vi "InitializeKeithley6485.vi"(8 "Error In":errorcluster, 10 "Keithley 6485":T1, 11 "VISA Resources":string[](array[string])) -> (0 "Error Out":errorcluster, 3 "Keithley 6485 Out":refnum<visa-resource-name>[](array[refnum]))   [LabVIEW 2012]
uses:
  Keithley6485Configuration.ctl
  libs/Keithley-6485/Public/Controls/FormatElement.ctl
  libs/Keithley-6485/Public/Controls/DataFormat.ctl
  libs/Keithley-6485/Keithley-6485.lvlib
  libs/LV-Utilities/LV-Utilities.lvlib
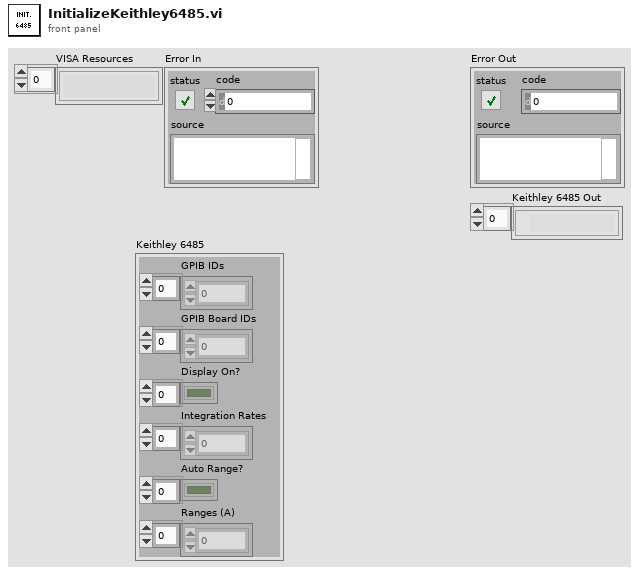
[diagram p1: front panel]
types:
  T1 = typedef "Keithley6485Configuration.ctl" = cluster{"GPIB IDs":u8[], "GPIB Board IDs":u8[], "Display On?":bool[], "Integration Rates":dbl[], "Auto Range?":bool[], "Ranges (A)":dbl[]}
  T2 = typedef "Keithley-6485.lvlib/DataFormat.ctl" = enum16{"ASCII", "Real", "32", "Sreal"}
  T3 = typedef "Keithley-6485.lvlib/FormatElement.ctl" = enum16{"Read", "Unit", "Time", "Status"}
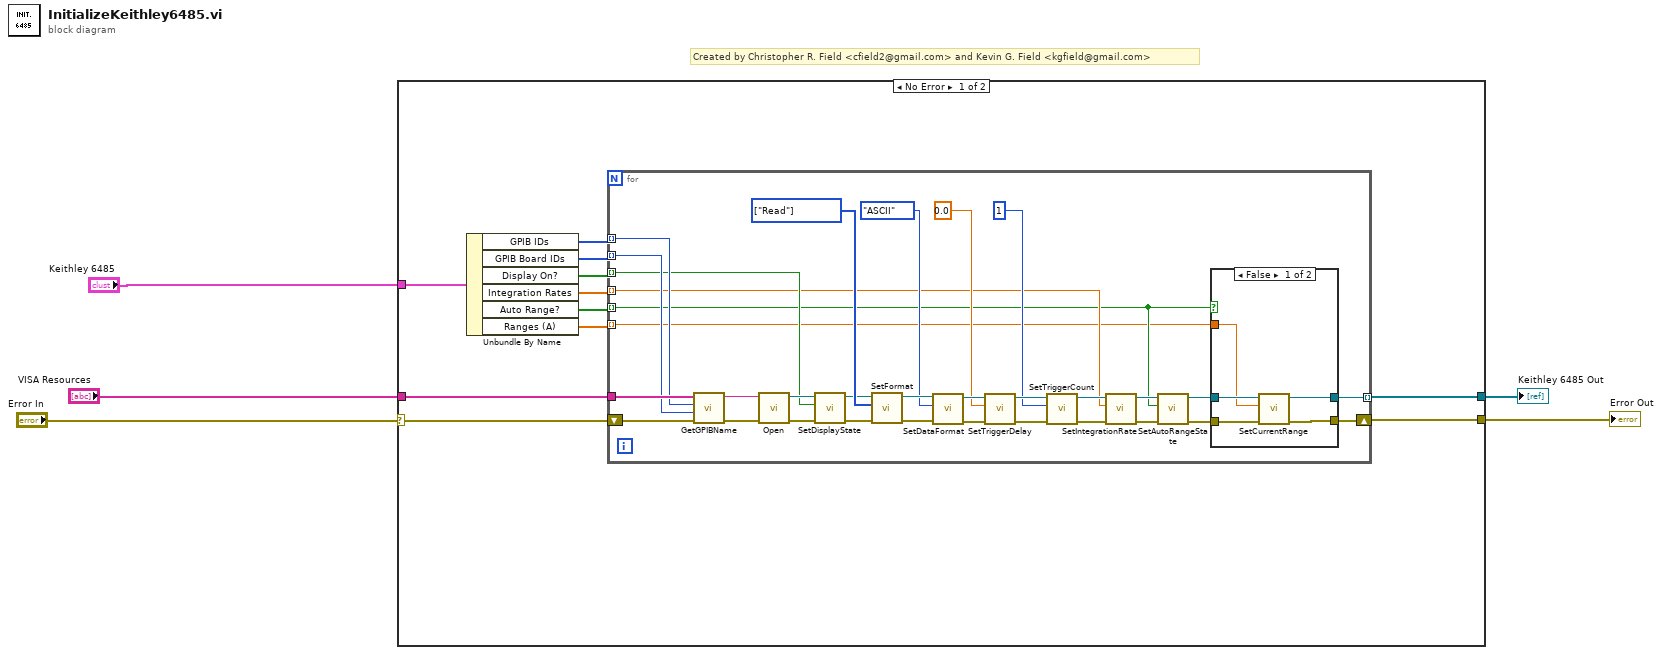
[diagram p0: block diagram]
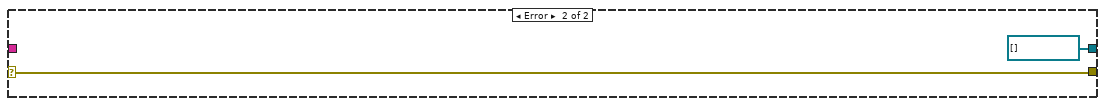
[diagram p3: hidden frame]
diagram:
  # "Created by Christopher R. Field <cfield2@gmail.com> and Kevin G. Field <kgfield@gmail.com>"
  n1 = case shown="No Error" "Error In" {
    selector: "Error In" -> [w6 w57]
    tunnel: "Keithley 6485" -> [w16 _]
    tunnel: "VISA Resources" -> [w9 _]
    tunnel: [w8 w57] -> w3
    tunnel: [w7 refnum<visa-resource-name>[] []] -> w2
    frame No Error {
      n2 = Unbundle By Name(w16) -> ("GPIB IDs"=w15:u8[], "GPIB Board IDs"=w14:u8[], "Display On?"=w13:bool[], "Integration Rates"=w12:dbl[], "Auto Range?"=w11:bool[], "Ranges (A)"=w10:dbl[])
      n3 = for {
        tunnel: w9 -> [w48]
        tunnel: w15 -> [w47] mode=indexing
        tunnel: w14 -> [w46] mode=indexing
        tunnel: w13 -> [w41] mode=indexing
        tunnel: [w19] -> w7 mode=indexing
        shift-right: [w18] -> w8
        shift-left: w6 -> [w24]
        tunnel: w12 -> [w23] mode=indexing
        tunnel: w11 -> [w22] mode=indexing
        tunnel: w10 -> [w17] mode=indexing
        w40 = T3[] [enum."Read"] items=["Read", "Unit", "Time", "Status"] ("Format Elements")
        n4 = call "GetGPIBName.vi"("Error In"=w24, "GPIB ID"=w46, "GPIB Board"=w47, "VISA Resource List"=w48) -> ("Error Out"=w45:errorcluster, "VISA GPIB Resource Name"=w44:string)  [unwired: 5 in, 1 out]
        n5 = call "Open.vi"("Error In"=w45, "Keithley 6485 In"=w44) -> ("Error Out"=w42:errorcluster, "Keithley 6485 Out"=w43:refnum<visa-resource-name>)  [unwired: 8 in]
        n6 = call "SetDisplayState.vi"("Error In"=w42, "Enabled?"=w41, "Keithley 6485 In"=w43) -> ("Error Out"=w38:errorcluster, "Keithley 6485 Out"=w39:refnum<visa-resource-name>)  [unwired: 7 in]
        n7 = call "SetFormat.vi"("Error In"=w38, "Format Elements"=w40, "Keithley 6485 In"=w39) -> ("Error Out"=w36:errorcluster, "Keithley 6485 Out"=w37:refnum<visa-resource-name>)  [unwired: 7 in]
        n8 = call "SetDataFormat.vi"("Error In"=w36, "Data Format"=DataFormat."ASCII", "Keithley 6485 In"=w37) -> ("Error Out"=w33:errorcluster, "Keithley 6485 Out"=w34:refnum<visa-resource-name>)  [unwired: 7 in]
        n9 = call "SetTriggerDelay.vi"("Error In"=w33, "Delay (sec)"=0.0, "Keithley 6485 In"=w34) -> ("Error Out"=w30:errorcluster, "Keithley 6485 Out"=w31:refnum<visa-resource-name>)  [unwired: 7 in]
        n10 = call "SetTriggerCount.vi"("Error In"=w30, "Count (1-3000)"=u16 1, "Keithley 6485 In"=w31) -> ("Error Out"=w27:errorcluster, "Keithley 6485 Out"=w28:refnum<visa-resource-name>)  [unwired: 7 in]
        n11 = call "SetIntegrationRate.vi"("Error In"=w27, "Integration Rate"=w23, "Keithley 6485 In"=w28) -> ("Error Out"=w25:errorcluster, "Keithley 6485 Out"=w26:refnum<visa-resource-name>)  [unwired: 7 in]
        n12 = call "SetAutoRangeState.vi"("Error In"=w25, "Enabled?"=w22, "Keithley 6485 In"=w26) -> ("Error Out"=w20:errorcluster, "Keithley 6485 Out"=w21:refnum<visa-resource-name>)  [unwired: 7 in]
        n13 = case shown="False" w22 {
          tunnel: w21 -> [w53 w55]
          tunnel: w20 -> [w50 w54]
          tunnel: [w52 w55] -> w19
          tunnel: [w51 w54] -> w18
          tunnel: w17 -> [w49 _]
          frame False {
            n14 = call "SetCurrentRange.vi"("Error In"=w50, "Expected Current (A)"=w49, "Keithley 6485 In"=w53) -> ("Error Out"=w51:errorcluster, "Keithley 6485 Out"=w52:refnum<visa-resource-name>)  [unwired: 7 in]
          }
          frame True {
          }
        }
      }
    }
    frame Error {
    }
  }
  "Error Out" <- w3
  "Keithley 6485 Out" <- w2
